vi "runtest Step Logic.vi"(7 "Do Not Print On Fail? (f)":bool, 8 "Step Results (empty)":T1, 11 "Stop on First Fail? (f)":bool) -> (0 "Save Data?":bool, 1 "Continue Testing?":bool, 2 "Not Aborted OR Error OR Fail?":bool, 3 "Not Pass OR Fail?":bool, 4 "Print?":bool)   [LabVIEW 2011]
uses:
  tests/Test Output.ctl
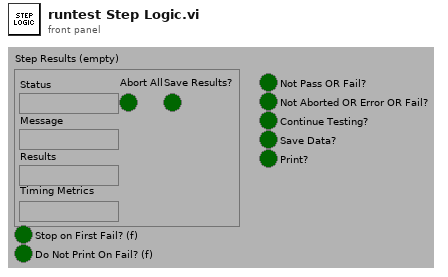
[diagram p1: front panel]
types:
  T1 = typedef "Test Output.ctl" = cluster{"Status":string, "Message":string, "Results":string, "Abort All":bool, "Save Results?":bool, "Timing Metrics":string}
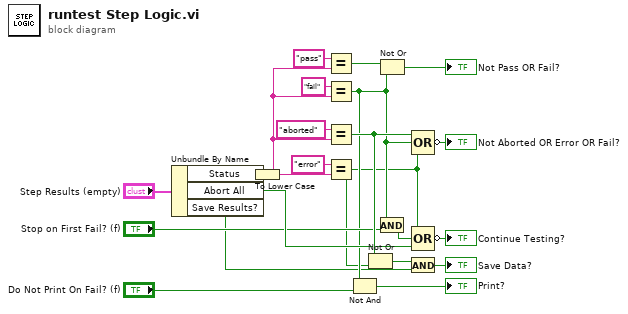
[diagram p0: block diagram]
diagram:
  n1 = Unbundle By Name("Step Results (empty)") -> ("Status"=w16:string, "Abort All"=w10:bool, "Save Results?"=w3:bool)
  n2 = To Lower Case(string=w16) -> (all lower case string=w15:string)
  n3 = Equal?(x="pass", y=w15) -> (x = y?=w18:bool)
  n4 = Equal?(x="fail", y=w15) -> (x = y?=w5:bool)
  n5 = Equal?(x="aborted", y=w15) -> (x = y?=w14:bool)
  n6 = Equal?(x="error", y=w15) -> (x = y?=w4:bool)
  n7 = Not And(1:"Do Not Print On Fail? (f)", 2:w5) -> (0:→"Print?":bool)
  n8 = Not Or(1:w4, 2:w14) -> (0:w2:bool)
  n9 = Not Or(1:w5, 2:w18) -> (0:→"Not Pass OR Fail?":bool)
  n10 = And(x=w5, y="Stop on First Fail? (f)") -> (x .and. y?=w11:bool)
  n11 = And(x=w2, y=w3) -> (x .and. y?=→"Save Data?":bool)
  n12 = Compound Arithmetic op=OR(w14, w5, w4) -> (invert →"Not Aborted OR Error OR Fail?":bool)
  n13 = Compound Arithmetic op=OR(w4, w11, w10) -> (invert →"Continue Testing?":bool)
